vi "ErrorHandler.Start.vi"(5 "Autoshutdown? (T)":bool=TRUE, 8 "error in (no error)":errorcluster, 11 "NewTemplate in":refnum<class "ErrorHandler.lvclass">) -> (0 "error out":errorcluster, 1 "StartupHandshake out":refnum<class "ModuleStartup.lvclass">, 2 "_TemplateModule":cluster{"Broadcasts":T1, "Broadcasts":T2}, 3 "NewTemplate out":refnum<class "ErrorHandler.lvclass">)   [LabVIEW 2024, in "ErrorHandler.lvclass"]
uses:
  ErrorHandler.lvclass/ErrorHandler.ctl
  ErrorHandler.lvclass
  C:/Git/JA/JQMH/RQMHCore/ModuleCore/Module.lvclass
  C:/Git/JA/JQMH/ModuleTemplates/ErrorHandler/ErrorHandler.lvclass
  RQMHCore/ModuleCore/Module.lvclass
  Stopped.ctl
  Broadcast Events--cluster.ctl
  RQMHCore/Shared/Died.ctl
  RQMHCore/Shared/ModuleShared.lvlib
  RQMHCore/ModuleCore/StandardBroadcasts.ctl
  RQMHCore/ModuleCore/Started.ctl
  RQMHCore/Startup/ModuleStartup.lvclass
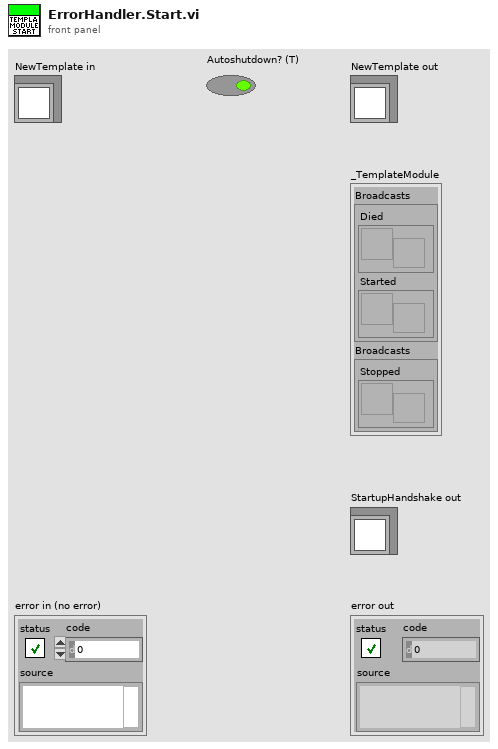
[diagram p1: front panel]
types:
  T1 = typedef "Module.lvclass/StandardBroadcasts.ctl" = cluster{"Died":refnum<user-event>, "Started":refnum<user-event>}
  T2 = typedef "ErrorHandler.lvclass/Broadcast Events--cluster.ctl" = cluster{"Stopped":refnum<user-event>}
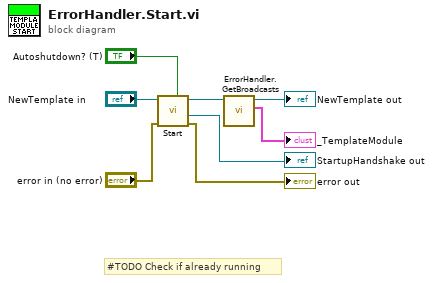
[diagram p0: block diagram]
diagram:
  # "#TODO Check if already running"
  n1 = call "Start.vi"("Autoshutdown? (T)"="Autoshutdown? (T)", "error in (no error)"="error in (no error)", "JQMHCore in"="NewTemplate in") -> ("error out"=→"error out":errorcluster, "StartupHandshake out"=→"StartupHandshake out":refnum<class "ModuleStartup.lvclass">, "JQMHCore out"=w4:refnum<class "ErrorHandler.lvclass">)  [unwired: 6 in]
  n2 = call "ErrorHandler.GetBroadcasts.vi"("NewTemplate in"=w4) -> ("TemplateModule"=→"_TemplateModule":cluster{"Broadcasts":T1, "Broadcasts":T2}, "NewTemplate out"=→"NewTemplate out":refnum<class "ErrorHandler.lvclass">)  [unwired: 9 in]
